vi "FanPressure2.vi"() -> ()   [LabVIEW 2023]
uses:
  <vilib>/drjdpowell/SQLite Library/SQL Connection/Connection.lvclass
  <vilib>/Instr/_visa.llb/VISA Find Search Mode.ctl
  <vilib>/drjdpowell/SQLite Library/SQL Connection/Open (path).vi
  <vilib>/Analysis/baseanly.llb/Mean (DBL).vi
  <vilib>/drjdpowell/SQLite Library/SQL Connection/Open (string).vi
  <vilib>/Instr/_visa.llb/VISA Configure Serial Port (Instr).vi
  <vilib>/drjdpowell/SQLite Library/SQL Connection/Execute SQL (No results).vi
  <vilib>/AdvancedString/Path To Command Line String.vi
  <vilib>/Analysis/NI_AALBase.lvlib
  <vilib>/drjdpowell/SQLite Library/SQLite.lvlib
panel:
  in  "Reset Plot 2":bool
  out "DC Power":bool
  in  "Message":string
  out "Receive Type":T1
  out "user event out":refnum<user-event>
  out "Table Name":string
  out "Table Created":bool
  out "time string":string
  out "date string":string
  out "SQLite Connection":refnum<class "Connection.lvclass">
  in  "View Data":bool
  in  "Reset Plot":bool
  in  "Write To Database":bool
  in  "Interval Time":u32=200
  out "Fan Speed":i32
  out "Fan Shunt Voltage":u16
  out "Fan Power":sgl
  out "Fan current":sgl
  out "Fan Voltage":sgl
  in  "Speed Control":enum32{"Values", "Paramters"}(tab)
  in  "Control Mode":enum32{"Auto", "Manual"}(radio)=enum."Manual"
  in  "Speed Setup":u16=2000 min=10 max=36 step=1
  in  "Output":sgl(knob) min=0 max=30 step=0.1 scale=0.0..30.0 scale format="%.1f"
  in  "Min Voltage":u32 max=12 step=1
  in  "Max Voltage":u32=30 min=12 max=36
  in  "Parameter Read Button":bool
  in  "Parameter Write Button":bool
  in  "Fan Speed At Full Output":u32
  in  "Fan Speed At 50% Output":u32
  in  "KD":sgl
  in  "KI":sgl=0.00015
  in  "KP":sgl=0.0024
  in  "Write Data":bool
  in  "Start Button":bool
  out "MCU":bool
  out "Serial Port":refnum<visa-resource-name>
  in  "stop":bool
  in  "Tab Control":enum32{"Readings", "Raw Data"}(tab)
  out "Waveform Chart 2":dbl[][](graph)
  out "Waveform Chart":sgl[][](graph)
  out "data":dynamicdata(graph) caption="Raw Data"
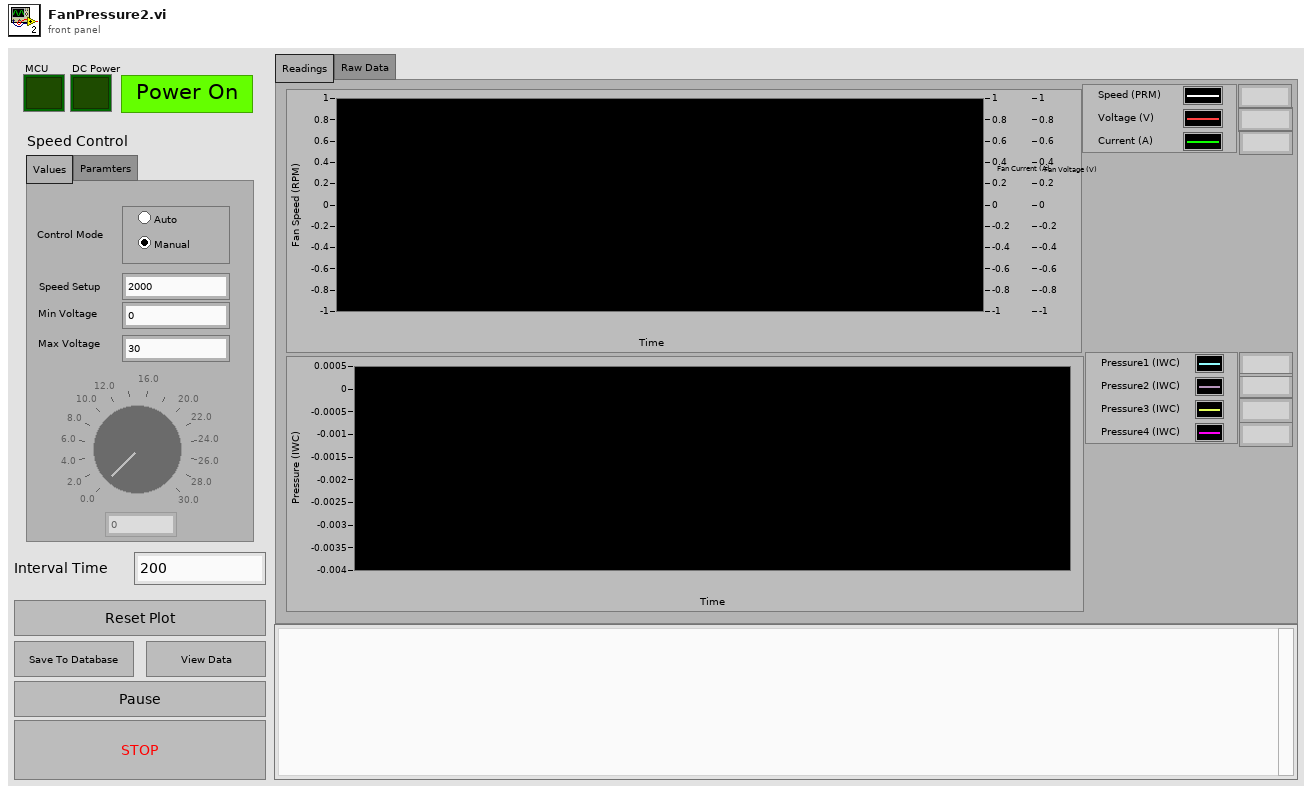
[diagram p1: front panel]
types:
  T1 = cluster{u8, u8, u8, u8, u16, u16, i16, i16, i16, i16, u16, u16, u16, u16, u16, u16, sgl, sgl, sgl, u32, u32, u8, u8, u8, u8}
  T2 = enum16{"New or existing", "Existing", "Read only"}
  T3 = enum8{"Enabled", "Disabled", "Disabled and Grayed Out"}
  T4 = enum32{"Invalid", "Standard", "Closed", "Hidden", "Minimized", "Maximized"}
  T5 = cluster{u32, "Fan current":sgl, "Fan current":sgl, "Fan current":sgl, "Fan Power":sgl, sgl, sgl, sgl, sgl, sgl, "Output":sgl, "Output":sgl}
  T6 = enum16{"big-endian, network order", "native, host order", "little-endian"}
  T7 = typedef "VISA Find Search Mode.ctl" = u32
  T8 = cluster{"y":u8, "y":u8, "y":u8, u8, u16, "Speed Setup":u16, u16, u16, "y":u8, "y":u8, "y":u8, "y":u8}
  T9 = cluster{"y":u8, "y":u8, "y":u8, "y":u8, "KP":sgl, "KI":sgl, "KD":sgl, "Fan Speed At 50% Output":u32, "Fan Speed At Full Output":u32, "y":u8, "y":u8, "y":u8, "y":u8}
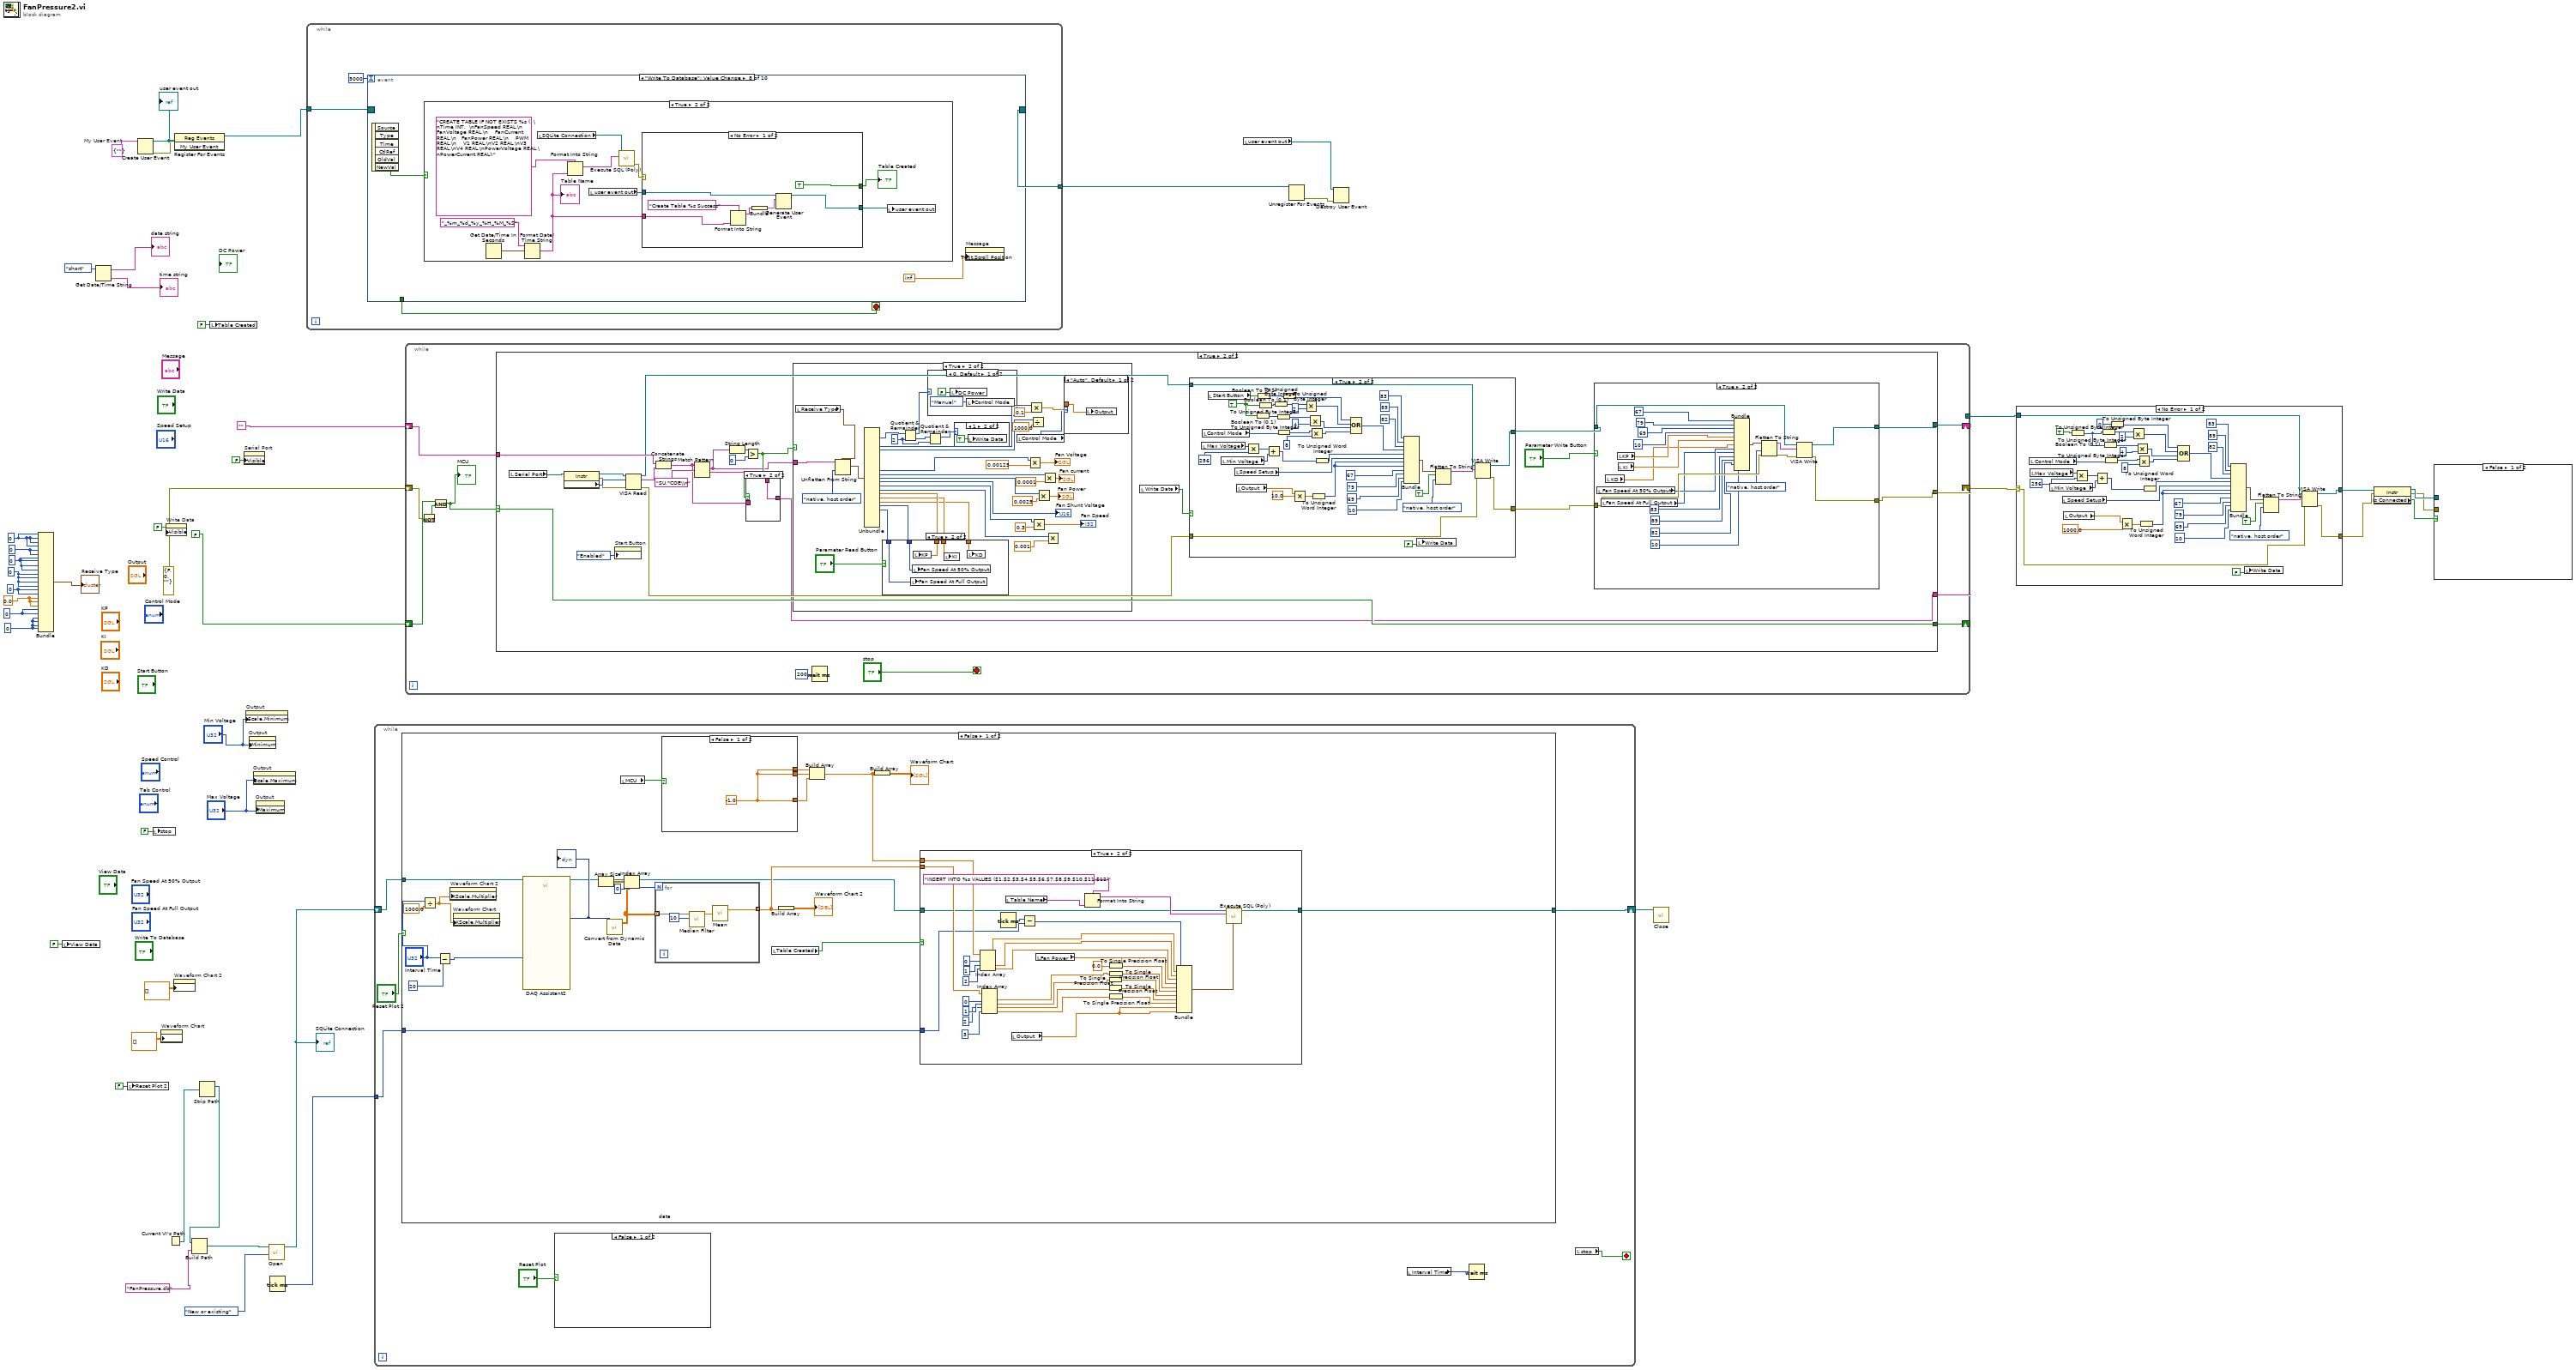
[diagram p0: block diagram]
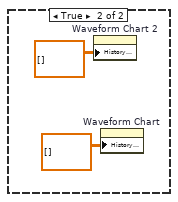
[diagram p2: hidden frame]
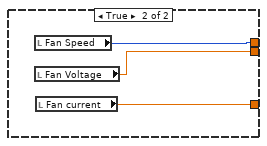
[diagram p4: hidden frame]
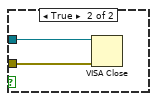
[diagram p6: hidden frame]
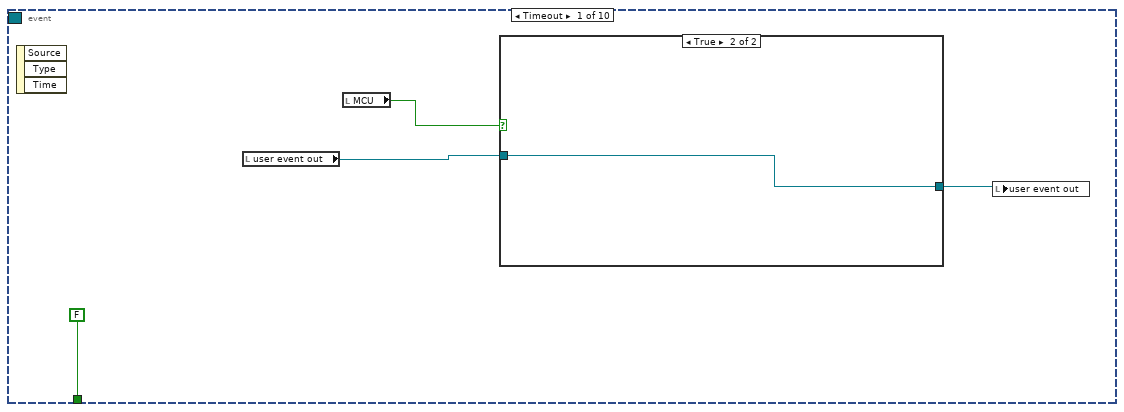
[diagram p8: hidden frame]
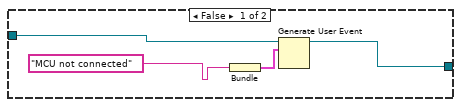
[diagram p9: hidden frame]
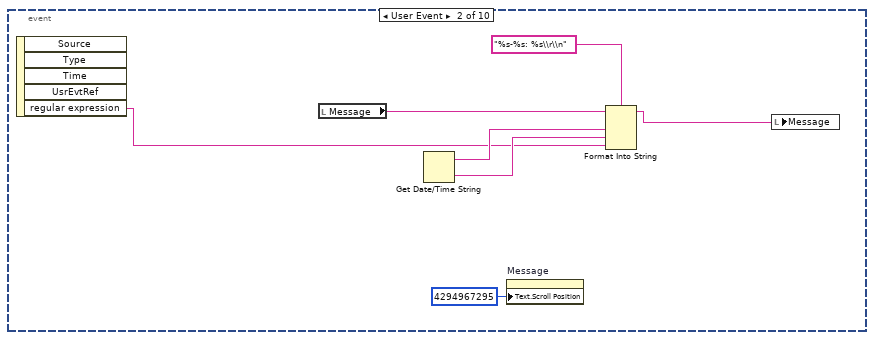
[diagram p10: hidden frame]
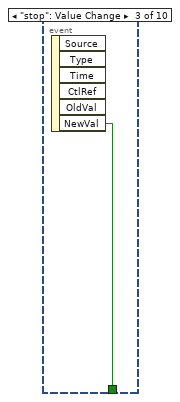
[diagram p11: hidden frame]
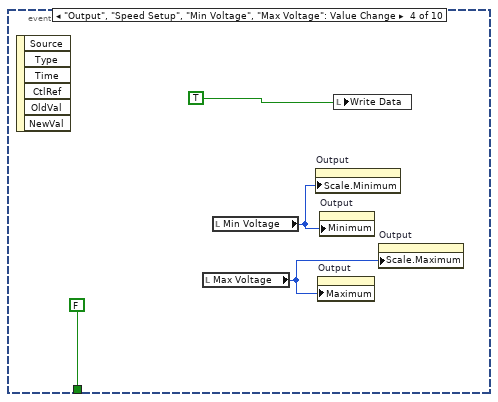
[diagram p12: hidden frame]
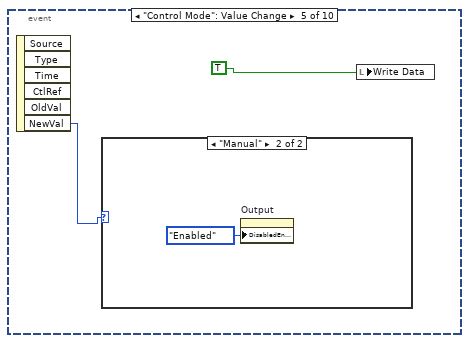
[diagram p13: hidden frame]
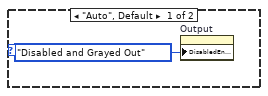
[diagram p14: hidden frame]
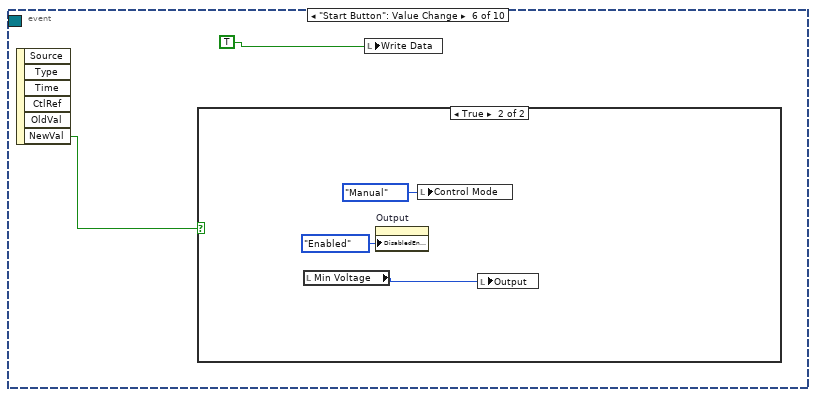
[diagram p15: hidden frame]
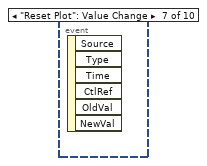
[diagram p17: hidden frame]
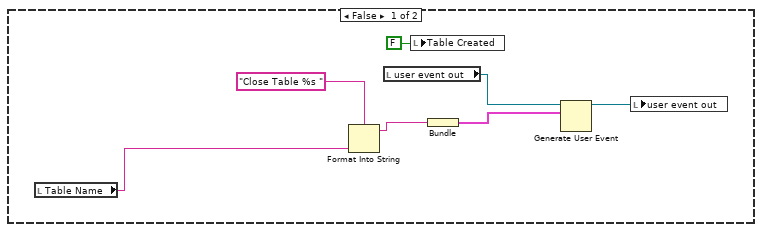
[diagram p18: hidden frame]
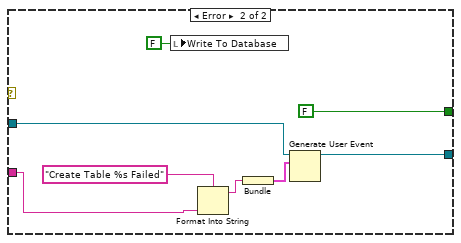
[diagram p19: hidden frame]
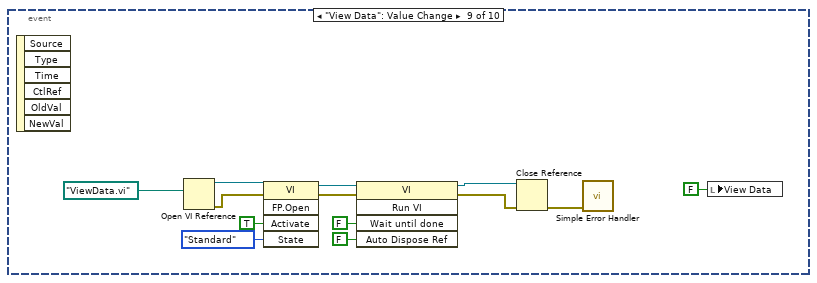
[diagram p20: hidden frame]
diagram:
  w3 = u32 0
  w4 = sgl 0.0
  w23 = cluster{"regular expression":string} {"regular expression"=""}  # My User Event
  w39 = u16 0
  w5 = u8 0
  w41 = i16 0
  w40 = u16 0
  w42 = u16 0
  w43 = u8 0
  n1 = Bundle(w43, w43, w43, w43, w42, w42, w41, w41, w41, w41, w39, w39, w39, w39, w40, w40, w4, w4, w4, w3, w3, w5, w5, w5, w5) -> (→"Receive Type":T1)  [unwired: 1 in]
  n2 = local write "View Data"(FALSE ("View Data")) -> ()
  n3 = Get Date/Time String(date format (0)=enum16{"short", "long", "abbreviated"}."short") -> (date string=→"date string":string, time string=→"time string":string)  [unwired: 2 in]
  n4 = local write "Reset Plot 2"(FALSE ("Reset Plot 2")) -> ()
  n5 = Create User Event(user event datatype=w23) -> (user event=w22:refnum<user-event>, error out=w20:errorcluster)  [unwired: 1 in]
  "user event out" <- w22
  n6 = local write "stop"(FALSE ("stop")) -> ()
  n7 = property on="Waveform Chart" class="WFChart (strict)"("History Data"=dbl[][] []) -> ()  [unwired: 2 in, 2 out]
  n8 = property on="Write Data" class="Bool (strict)"("Visible"=FALSE) -> ()  [unwired: 2 in, 2 out]
  n9 = Current VI's Path() -> (path=w14:path)
  n10 = property on="Waveform Chart 2" class="WFChart (strict)"("History Data"=dbl[][] []) -> ()  [unwired: 2 in, 2 out]
  n11 = register-events(error in=w20, w22) -> (reference out=w21:refnum<event-registration>)  [unwired: 1 in, 1 out]
  n12 = Strip Path(path=w14) -> (stripped path=w13:path)  [unwired: 1 out]
  n13 = Build Path(base path=w13, name or relative path="FanPressure.db" ("db file")) -> (appended path=w15:path)
  n14 = local write "Table Created"(FALSE ("Table Created")) -> ()
  n15 = property on="Serial Port" class="VISAName"("Visible"=FALSE) -> ()  [unwired: 2 in, 2 out]
  n16 = property on="Output" class="Knob (strict)"("Scale.Minimum"="Min Voltage") -> ()  [unwired: 2 in, 2 out]
  n17 = property on="Output" class="Knob (strict)"("Minimum"="Min Voltage") -> ()  [unwired: 2 in, 2 out]
  n18 = property on="Output" class="Knob (strict)"("Scale.Maximum"="Max Voltage") -> ()  [unwired: 2 in, 2 out]
  n19 = property on="Output" class="Knob (strict)"("Maximum"="Max Voltage") -> ()  [unwired: 2 in, 2 out]
  n20 = call-poly <vilib>:"Open.vi"("File Option"=T2."New or existing", "db file"=w15) -> ("SQLite Connection"=w12:refnum<class "Connection.lvclass">)  [unwired: 8 in, 1 out]
  "SQLite Connection" <- w12
  n21 = Tick Count (ms)() -> (millisecond timer value=w9:u32)
  n22 = while {
    tunnel: w21 -> [w50]
    tunnel: [w49] -> w19
    stop <- w51 stop-if-true
    n23 = event shown="[7] \"Write To Database\": Value Change" {
      selector: w50 -> [_ _ _ _ _ _ _ _ _ _]
      dyn-events: [_ _ _ _ _ _ _ _ _ _] -> w49
      timeout: 5000 -> [_ _ _ _ _ _ _ _ _ _]
      tunnel: [FALSE ("NewVal") _ w68 FALSE ("NewVal") _ _ _ _ _ _] -> w51
      event Timeout {
        n24 = event-data() -> ()  [unwired: 1 in, 3 out]
        n25 = local read "user event out"() -> (w54:refnum<user-event>)
        n26 = local read "MCU"() -> (w52:bool)
        n27 = case shown="True" w52 {
          tunnel: w54 -> [w57 w60]
          tunnel: [w58 w60] -> w53
          frame False {
            n28 = Bundle("format string"="MCU not connected") -> (w59:cluster{"format string":string})  [unwired: 1 in]
            n29 = Generate User Event(user event=w57, event data cluster=w59) -> (user event out=w58:refnum<user-event>)  [unwired: 2 in, 1 out]
          }
          frame True {
          }
        }
        n30 = local write "user event out"(w53) -> ()
      }
      event User Event {
        n31 = event-data() -> ("regular expression"=w62:string)  [unwired: 1 in, 4 out]
        n32 = local read "Message"() -> (w67:string)
        n33 = Get Date/Time String() -> (date string=w66:string, time string=w65:string)  [unwired: 3 in]
        n34 = property on="Message" class="Str"("Text.Scroll Position"=u32 4294967295) -> ()  [unwired: 2 in, 2 out]
        n35 = Format Into String(format string="%s-%s: %s\\r\\n", initial string=w67, w66, w65, w62) -> (resulting string=w64:string)  [unwired: 1 in, 1 out]
        n36 = local write "Message"(w64) -> ()
      }
      event "stop": Value Change {
        n37 = event-data() -> ("NewVal"=w68:bool)  [unwired: 1 in, 5 out]
      }
      event "Output", "Speed Setup", "Min Voltage", "Max Voltage": Value Change {
        n38 = event-data() -> ()  [unwired: 1 in, 6 out]
        n39 = local read "Max Voltage"() -> (w69:u32)
        n40 = local read "Min Voltage"() -> (w70:u32)
        n41 = property on="Output" class="Knob (strict)"("Scale.Minimum"=w70) -> ()  [unwired: 2 in, 2 out]
        n42 = property on="Output" class="Knob (strict)"("Maximum"=w69) -> ()  [unwired: 2 in, 2 out]
        n43 = property on="Output" class="Knob (strict)"("Minimum"=w70) -> ()  [unwired: 2 in, 2 out]
        n44 = local write "Write Data"(TRUE ("Write Data")) -> ()
        n45 = property on="Output" class="Knob (strict)"("Scale.Maximum"=w69) -> ()  [unwired: 2 in, 2 out]
      }
      event "Control Mode": Value Change {
        n46 = event-data() -> ("NewVal"=w73:enum32{"Auto", "Manual"})  [unwired: 1 in, 5 out]
        n47 = case shown="\"Manual\"" w73 {
          frame "Auto", Default {
            n48 = property on="Output" class="Knob (strict)"("DisabledEnum"=T3."Disabled and Grayed Out" ("Disabled")) -> ()  [unwired: 2 in, 2 out]
          }
          frame "Manual" {
            n49 = property on="Output" class="Knob (strict)"("DisabledEnum"=T3."Enabled" ("Disabled")) -> ()  [unwired: 2 in, 2 out]
          }
        }
        n50 = local write "Write Data"(TRUE ("Write Data")) -> ()
      }
      event "Start Button": Value Change {
        n51 = event-data() -> ("NewVal"=w77:bool)  [unwired: 1 in, 5 out]
        n52 = case shown="True" w77 {
          frame False {
          }
          frame True {
            n53 = local read "Min Voltage"() -> (w80:u32)
            n54 = property on="Output" class="Knob (strict)"("DisabledEnum"=T3."Enabled" ("Disabled")) -> ()  [unwired: 2 in, 2 out]
            n55 = local write "Control Mode"(enum32{"Auto", "Manual"}."Manual" ("Control Mode")) -> ()
            n56 = local write "Output"(w80) -> ()
          }
        }
        n57 = local write "Write Data"(TRUE ("Write Data")) -> ()
      }
      event "Reset Plot": Value Change {
        n58 = event-data() -> ()  [unwired: 1 in, 6 out]
      }
      event "Write To Database": Value Change {
        n59 = event-data() -> ("NewVal"=w83:bool)  [unwired: 1 in, 5 out]
        n60 = case shown="True" w83 {
          frame False {
            n61 = local read "Table Name"() -> (w89:string)
            n62 = Format Into String(format string="Close Table %s ", w89) -> (resulting string=w86:string)  [unwired: 2 in, 1 out]
            n63 = local read "user event out"() -> (w87:refnum<user-event>)
            n64 = local write "Table Created"(FALSE ("Table Created")) -> ()
            n65 = Bundle(w86) -> (w85:cluster{string})  [unwired: 1 in]
            n66 = Generate User Event(user event=w87, event data cluster=w85) -> (user event out=w84:refnum<user-event>)  [unwired: 2 in, 1 out]
            n67 = local write "user event out"(w84) -> ()
          }
          frame True {
            n68 = Get Date/Time In Seconds() -> (seconds since 1Jan1904=w99:timestamp)
            n69 = Format Date/Time String(time format string (%c)="_%m_%d_%y_%H_%M_%S", seconds (now)=w99) -> (date/time string=w91:string)  [unwired: 1 in]
            "Table Name" <- w91
            n70 = local read "SQLite Connection"() -> (w100:refnum<class "Connection.lvclass">)
            n71 = Format Into String(format string="CREATE TABLE IF NOT EXISTS %s (  \nTime INT,  \nFanSpeed REAL,\n    FanVoltage REAL,\n    FanCurrent REAL,\n   FanPower REAL,\n    PWM REAL,\n    V1 REAL,\nV2 REAL,\nV3 REAL,\nV4 REAL,\nPowerVoltage REAL,\nPowerCurrent REAL);" ("SQL"), w91) -> (resulting string=w96:string)  [unwired: 2 in, 1 out]
            n72 = local read "user event out"() -> (w93:refnum<user-event>)
            n73 = call-poly <vilib>:"Execute SQL (Poly).vi"("SQL"=w96, "SQLite Connection in"=w100) -> ("error out"=w95:errorcluster)  [unwired: 8 in, 1 out]
            n74 = case shown="No Error" w95 {
              tunnel: [TRUE ("Table Created") FALSE ("Table Created")] -> w94
              tunnel: w93 -> [w101 w110]
              tunnel: [w102 w109] -> w92
              tunnel: w91 -> [w103 w108]
              frame No Error {
                n75 = Format Into String(format string="Create Table %s Success", w103) -> (resulting string=w106:string)  [unwired: 2 in, 1 out]
                n76 = Bundle(w106) -> (w105:cluster{string})  [unwired: 1 in]
                n77 = Generate User Event(user event=w101, event data cluster=w105) -> (user event out=w102:refnum<user-event>)  [unwired: 2 in, 1 out]
              }
              frame Error {
                n78 = local write "Write To Database"(FALSE ("Write To Database")) -> ()
                n79 = Format Into String(format string="Create Table %s Failed", w108) -> (resulting string=w113:string)  [unwired: 2 in, 1 out]
                n80 = Bundle(w113) -> (w112:cluster{string})  [unwired: 1 in]
                n81 = Generate User Event(user event=w110, event data cluster=w112) -> (user event out=w109:refnum<user-event>)  [unwired: 2 in, 1 out]
              }
            }
            "Table Created" <- w94
            n82 = local write "user event out"(w92) -> ()
          }
        }
        n83 = property on="Message" class="Str"("Text.Scroll Position"=inf) -> ()  [unwired: 2 in, 2 out]
      }
      event "View Data": Value Change {
        n84 = event-data() -> ()  [unwired: 1 in, 6 out]
        n85 = Open VI Reference(vi path=path "ViewData.vi") -> (vi reference=w126:refnum<vi>, error out=w119:errorcluster)  [unwired: 5 in]
        n86 = invoke class="VI" method="FP.Open"(reference=w126, error in=w119, "Activate"=TRUE ("Activate?"), "State"=T4."Standard") -> (reference out=w123:refnum<vi>, error out=w122:errorcluster)  [unwired: 1 in, 3 out]
        n87 = invoke class="VI" method="Run VI"(reference=w123, error in=w122, "Wait until done"=FALSE ("Wait Until Done"), "Auto Dispose Ref"=FALSE ("Auto Dispose Reference")) -> (reference out=w118:refnum<vi>, error out=w117:errorcluster)  [unwired: 1 in, 3 out]
        n88 = Close Reference(reference=w118, error in (no error)=w117) -> (error out=w116:errorcluster)
        n89 = call <vilib>:"Simple Error Handler.vi"("error in (no error)"=w116) -> ()  [unwired: 4 in, 5 out]
        n90 = local write "View Data"(FALSE ("View Data")) -> ()
      }
      event "Message": Value Change {
        n91 = event-data() -> ()  [unwired: 1 in, 6 out]
      }
    }
  }
  n92 = while {
    shift-right: [w133] -> w11
    shift-left: w12 -> [w132]
    tunnel: w9 -> [w131]
    stop <- w135 stop-if-true
    n93 = case shown="False" "Reset Plot 2" {
      tunnel: [w140 w202] -> w133
      tunnel: w132 -> [w139 w202]
      tunnel: w131 -> [w138 _]
      frame False {
        n94 = Divide(x="Interval Time", y=1000.0) -> (x/y=w149:dbl)
        n95 = Subtract(x="Interval Time", y=u32 20) -> (x-y=w157:u32)
        n96 = property on="Waveform Chart 2" class="WFChart (strict)"("XScale.Multiplier"=w149) -> ()  [unwired: 2 in, 2 out]
        n97 = property on="Waveform Chart" class="WFChart (strict)"("XScale.Multiplier"=w149) -> ()  [unwired: 2 in, 2 out]
        n98 = call "DAQ Assistant2"("number of samples"=w157) -> ("data"=w159:dynamicdata)  [unwired: 16 in, 2 out]
        "data" <- w159
        n99 = call "Convert from Dynamic Data"("Dynamic Data Type"=w159) -> ("Array"=w156:dbl[][])  [unwired: 3 in]
        n100 = Array Size(array=w156) -> (size(s)=w155:i32[])
        n101 = local read "MCU"() -> (w148:bool)
        n102 = Index Array(array=w155, index=0) -> (element=w153:i32)
        n103 = for {
          N: w153 -> [_]
          tunnel: w156 -> [w201] mode=indexing
          tunnel: [w198] -> w143 mode=indexing
          n104 = call <vilib>:"Median Filter.vi"("left rank"=10, "X"=w201) -> ("Filtered X"=w199:dbl[])  [unwired: 8 in, 1 out]
          n105 = call-poly <vilib>:"Mean.vi"("X"=w199) -> ("mean"=w198:dbl)  [unwired: 1 out]
        }
        n106 = case shown="False" w148 {
          tunnel: [w194 w197] -> w147
          tunnel: [w194 w196] -> w146
          tunnel: [w194 w195] -> w145
          frame False {
            w194 = sgl -1.0 ("Fan current")
          }
          frame True {
            n107 = local read "Fan Speed"() -> (w195:i32)
            n108 = local read "Fan Voltage"() -> (w196:sgl)
            n109 = local read "Fan current"() -> (w197:sgl)
          }
        }
        n110 = local read "Table Created"() -> (w141:bool)
        n111 = Build Array(w143) -> (→"Waveform Chart 2":dbl[][])
        n112 = Build Array(w145, w146, w147) -> (w142:sgl[])
        n113 = Build Array(w142) -> (→"Waveform Chart":sgl[][])
        n114 = case shown="True" w141 {
          tunnel: w143 -> [_ w189]
          tunnel: w142 -> [_ w193]
          tunnel: w139 -> [w160 w176]
          tunnel: [w160 w175] -> w140
          tunnel: w138 -> [_ w164]
          frame False {
          }
          frame True {
            n115 = Index Array(array=w193, index #1=0 ("index"), index #2=1 ("index"), index #3=2 ("index")) -> (element #1=w184:sgl, element #2=w183:sgl, element #3=w182:sgl)
            n116 = Index Array(array=w189, index #1=0 ("index"), index #2=1 ("index"), index #3=2 ("index"), index #4=3 ("index")) -> (element #1=w168:dbl, element #2=w170:dbl, element #3=w172:dbl, element #4=w174:dbl)
            n117 = Tick Count (ms)() -> (millisecond timer value=w165:u32)
            n118 = local read "Table Name"() -> (w178:string)
            n119 = local read "Output"() -> (w161:sgl)
            n120 = Subtract(x=w165, y=w164) -> (x-y=w163:u32)
            n121 = local read "Fan Power"() -> (w181:sgl)
            n122 = Format Into String(format string="INSERT INTO %s VALUES ($1,$2,$3,$4,$5,$6,$7,$8,$9,$10,$11,$12)" ("SQL"), w178) -> (resulting string=w177:string)  [unwired: 2 in, 1 out]
            n123 = To Single Precision Float(number=w170) -> (single precision float=w169:sgl)
            n124 = To Single Precision Float(number=w172) -> (single precision float=w171:sgl)
            n125 = To Single Precision Float(number=sgl 0.0) -> (single precision float=w166:sgl)
            n126 = To Single Precision Float(number=w168) -> (single precision float=w167:sgl)
            n127 = To Single Precision Float(number=w174) -> (single precision float=w173:sgl)
            n128 = Bundle(w163, "Fan current"=w184, "Fan current"=w183, "Fan current"=w182, "Fan Power"=w181, w166, w167, w169, w171, w173, "Output"=w161, "Output"=w161) -> (w180:T5)  [unwired: 1 in]
            n129 = call-poly <vilib>:"Execute SQL (Poly).vi"("Parameter(s)"=w180, "SQL"=w177, "SQLite Connection in"=w176) -> ("SQLite Connection"=w175:refnum<class "Connection.lvclass">)  [unwired: 7 in, 1 out]
          }
        }
      }
      frame True {
      }
    }
    n130 = case shown="False" "Reset Plot" {
      frame False {
      }
      frame True {
        n131 = property on="Waveform Chart 2" class="WFChart (strict)"("History Data"=dbl[][] []) -> ()  [unwired: 2 in, 2 out]
        n132 = property on="Waveform Chart" class="WFChart (strict)"("History Data"=dbl[][] []) -> ()  [unwired: 2 in, 2 out]
      }
    }
    n133 = local read "Interval Time"() -> (w134:u32)
    n134 = Wait (ms)(milliseconds to wait=w134) -> ()  [unwired: 1 out]
    n135 = local read "stop"() -> (w135:bool)
  }
  n136 = while {
    shift-right: [w212] -> _
    shift-left: FALSE -> [w210]
    shift-right: [w211] -> w36
    shift-left: errorcluster {"status"=FALSE, "code"=0, "source"=""} ("error in (no error)") -> [w206]
    tunnel: [w208] -> w37
    shift-right: [w205] -> _
    shift-left: "" -> [w204]
    stop <- "stop" stop-if-true
    n137 = Not(x=w206) -> (.not. x?=w209:bool)
    n138 = And(x=w210, y=w209) -> (x .and. y?=w203:bool)
    "MCU" <- w203
    n139 = case shown="True" w203 {
      selector: w203 -> [w216 w270]
      tunnel: [w220 w270] -> w212
      tunnel: [w219 w263] -> w211
      tunnel: [w218 w265] -> w208
      tunnel: w204 -> [_ w275]
      tunnel: ["" w259] -> w205
      frame False {
        w223 = T7 2 items=["Canonical Names Only"=0, "Aliases Only"=2, "Include Matching Aliases"=3, "Include All Aliases"=4] ("Search Mode")
        n140 = local write "Start Button"(w216) -> ()
        n141 = local write "DC Power"(FALSE ("DC Power")) -> ()
        n142 = property on="Start Button" class="Bool (strict)"("DisabledEnum"=T3."Disabled and Grayed Out" ("Disabled")) -> ()  [unwired: 2 in, 2 out]
        n143 = VISA Find Resource(10:w223, 11:"ASRL[0-9]*::?*INSTR" ("expression (\"?*\")")) -> (0:w221:errorcluster, 3:w222:string[])  [unwired: 1 in, 1 out]
        n144 = for {
          tunnel: w222 -> [w229] mode=indexing
          tunnel: w221 -> [w241]
          tunnel: [w233] -> w220
          tunnel: [w226] -> w219
          tunnel: [w225] -> w218
          stop <- w232 stop-if-true
          n145 = call-poly "VISA Configure Serial Port"("VISA resource name"=w229, "baud rate (9600)"=u32 115200, "error in (no error)"=w241) -> ("VISA resource name out"=w228:refnum<visa-resource-name>, "error out"=w240:errorcluster)  [unwired: 11 in]
          n146 = property class="Instr"(reference=w228, error in=w240) -> (reference out=w231:refnum<visa-resource-name>, error out=w237:errorcluster, "Intf Inst Name"=w239:string)
          n147 = Search and Replace String(case sensitive?=TRUE ("ignore case? (F)"), input string=w239, search string="CP210x", error in=w237) -> (number of replacements=w235:i32, error out=w227:errorcluster)  [unwired: 4 in, 2 out]
          n148 = Greater?(x=w235, y=0) -> (0:w233:bool)
          n149 = case shown="True" w233 {
            selector: w233 -> [w245 w256]
            tunnel: [w245 w256] -> w232
            tunnel: w231 -> [w242 w254]
            tunnel: w227 -> [w244 w255]
            tunnel: [w243 w248] -> w226
            tunnel: [w242 w250] -> w225
            frame False {
              n150 = VISA Close(VISA resource name=w242, error in (no error)=w244) -> (error out=w243:errorcluster)
            }
            frame True {
              n151 = VISA Close(VISA resource name=w254, error in (no error)=w255) -> (error out=w247:errorcluster)
              n152 = call-poly "VISA Configure Serial Port"("VISA resource name"=w254, "baud rate (9600)"=u32 115200, "error in (no error)"=w247) -> ("VISA resource name out"=w252:refnum<visa-resource-name>, "error out"=w246:errorcluster)  [unwired: 11 in]
              n153 = VISA Open(error in (no error)=w246, VISA resource name=w252) -> (VISA resource name=w251:refnum<visa-resource-name>, error out=w249:errorcluster)  [unwired: 3 in]
              n154 = VISA Flush I/O Buffer(VISA resource name=w251, error in (no error)=w249) -> (VISA resource name out=w250:refnum<visa-resource-name>, error out=w248:errorcluster)  [unwired: 1 in]
              "Serial Port" <- w250
            }
          }
        }
      }
      frame True {
        n155 = local read "Serial Port"() -> (w280:refnum<visa-resource-name>)
        n156 = property class="Instr"(reference=w280) -> (reference out=w278:refnum<visa-resource-name>, error out=w277:errorcluster, "Serial Settings:Number of Bytes at Serial Port"=w279:u32)  [unwired: 1 in]
        n157 = property on="Start Button" class="Bool (strict)"("DisabledEnum"=T3."Enabled" ("Disabled")) -> ()  [unwired: 2 in, 2 out]
        n158 = VISA Read(VISA resource name=w278, byte count=w279, error in (no error)=w277) -> (VISA resource name out=w271:refnum<visa-resource-name>, read buffer=w276:string, error out=w267:errorcluster)  [unwired: 1 out]
        n159 = Concatenate Strings(w275, w276) -> (w258:string)
        n160 = Match Pattern(string=w258, regular expression="SU.*COE\\n") -> (match substring=w260:string, after substring=w257:string)  [unwired: 1 in, 2 out]
        n161 = String Length(string=w260) -> (length=w273:i32)
        n162 = Greater?(x=w273, y=0) -> (0:w261:bool)
        n163 = case shown="True" w261 {
          tunnel: [w281 w282] -> w259
          tunnel: w257 -> [_ w282]
          tunnel: w258 -> [w281 _]
          frame False {
          }
          frame True {
          }
        }
        n164 = case shown="True" w261 {
          tunnel: w260 -> [_ w387]
          frame False {
          }
          frame True {
            w353 = u8 2 ("y")
            n165 = local read "Receive Type"() -> (w364:T1)
            n166 = Unflatten From String(type=w364, binary string=w387, byte order (0:big-endian, network order)=T6."native, host order") -> (value=w385:T1)  [unwired: 2 in, 2 out]
            n167 = Unbundle(w385) -> (w355:u8, w384:u16, w382:u16, w379:u16, w375:u16, w373:u16, →"Fan Shunt Voltage":u16, w369:u16, w367:u16, w362:sgl, w361:sgl, w360:sgl, w359:u32, w358:u32)  [unwired: 11 out]
            n168 = case shown="True" "Parameter Read Button" {
              tunnel: w362 -> [_ w397]
              tunnel: w361 -> [_ w396]
              tunnel: w360 -> [_ w395]
              tunnel: w359 -> [_ w394]
              tunnel: w358 -> [_ w393]
              frame False {
              }
              frame True {
                n169 = local write "Fan Speed At Full Output"(w393) -> ()
                n170 = local write "Fan Speed At 50% Output"(w394) -> ()
                n171 = local write "KP"(w397) -> ()
                n172 = local write "KI"(w396) -> ()
                n173 = local write "KD"(w395) -> ()
              }
            }
            n174 = Quotient & Remainder(x=w355, y=w353) -> (x-y*floor(x/y)=w356:u8, floor(x/y)=w354:u8)
            n175 = case shown="0, Default" w356 {
              frame 0, Default {
                n176 = local write "DC Power"(FALSE ("DC Power")) -> ()
                n177 = local write "Control Mode"(enum32{"Auto", "Manual"}."Manual" ("Control Mode")) -> ()
              }
              frame 1 {
                n178 = local write "DC Power"(TRUE ("DC Power")) -> ()
              }
            }
            n179 = Quotient & Remainder(x=w354, y=w353) -> (x-y*floor(x/y)=w352:u8)  [unwired: 1 out]
            n180 = case shown="1" w352 {
              frame 0, Default {
              }
              frame 1 {
                n181 = local write "Write Data"(TRUE ("Write Data")) -> ()
              }
            }
            n182 = local read "Control Mode"() -> (w357:enum32{"Auto", "Manual"})
            n183 = Multiply(x=w379, y=0.00125) -> (x*y=→"Fan Voltage":dbl)
            n184 = Multiply(x=w384, y=0.1) -> (x*y=w365:dbl)
            n185 = Divide(x=w382, y=1000.0) -> ()  [unwired: 1 out]
            n186 = Multiply(x=w369, y=0.3) -> (x*y=→"Fan Speed":dbl)
            n187 = Multiply(x=w373, y=0.0025) -> (x*y=→"Fan Power":dbl)
            n188 = Multiply(x=w375, y=0.0001) -> (x*y=→"Fan current":dbl)
            n189 = Multiply(x=w367, y=0.001) -> ()  [unwired: 1 out]
            n190 = case shown="\"Auto\", Default" w357 {
              tunnel: w365 -> [w392 _]
              frame "Auto", Default {
                n191 = local write "Output"(w392) -> ()
              }
              frame "Manual" {
              }
            }
          }
        }
        n192 = local read "Write Data"() -> (w268:bool)
        n193 = case shown="True" w268 {
          tunnel: w271 -> [w307 w351]
          tunnel: [w307 w350] -> w266
          tunnel: w267 -> [w306 w349]
          tunnel: [w306 w348] -> w264
          frame False {
          }
          frame True {
            w314 = TRUE ("Boolean")
            n194 = local read "Max Voltage"() -> (w313:u32)
            n195 = local read "Control Mode"() -> (w315:enum32{"Auto", "Manual"})
            n196 = local read "Start Button"() -> (w344:bool)
            n197 = local read "Min Voltage"() -> (w310:u32)
            n198 = local read "Speed Setup"() -> (w328:u16)
            n199 = local read "Output"() -> (w326:sgl)
            n200 = Multiply(x=w313, y=u32 256) -> (x*y=w311:u32)
            n201 = Boolean To (0,1)(Boolean=w314) -> (0, 1=w343:i16)
            n202 = Boolean To (0,1)(Boolean=w344) -> (0, 1=w345:i16)
            n203 = Boolean To (0,1)(Boolean=w314) -> (0, 1=w346:i16)
            n204 = Add(x=w311, y=w310) -> (x+y=w309:u32)
            n205 = To Unsigned Byte Integer(number=w346) -> (unsigned 8bit integer=w338:u8)
            n206 = To Unsigned Byte Integer(number=w343) -> (unsigned 8bit integer=w335:u8)
            n207 = To Unsigned Byte Integer(number=w315) -> (unsigned 8bit integer=w334:u8)
            n208 = To Unsigned Byte Integer(number=w345) -> (unsigned 8bit integer=w342:u8)
            n209 = Multiply(x=w326, y=sgl 10.0) -> (x*y=w325:sgl)
            n210 = Multiply(x=w338, y=u8 2) -> (x*y=w336:u8)
            n211 = Multiply(x=w335, y=u8 4) -> (x*y=w330:u8)
            n212 = Multiply(x=w334, y=u8 8 ("x")) -> (x*y=w332:u8)
            n213 = To Unsigned Word Integer(number=w325) -> (unsigned 16bit integer=w324:u16)
            n214 = To Unsigned Word Integer(number=w309) -> (unsigned 16bit integer=w329:u16)
            n215 = Compound Arithmetic op=OR(w342, w336, w330, w332) -> (w341:u8)
            n216 = Bundle("y"=u8 83, "y"=u8 89, "y"=u8 82, w341, w329, "Speed Setup"=w328, w324, w324, "y"=u8 67, "y"=u8 79, "y"=u8 69, "y"=u8 10) -> (w316:T8)  [unwired: 1 in]
            n217 = local write "Write Data"(FALSE ("Write Data")) -> ()
            n218 = Flatten To String(anything=w316, prepend array or string size? (T)=TRUE, byte order (0:big-endian, network order)=T6."native, host order") -> (data string=w308:string)  [unwired: 1 in, 2 out]
            n219 = VISA Write(VISA resource name=w351, write buffer=w308, error in (no error)=w349) -> (VISA resource name out=w350:refnum<visa-resource-name>, error out=w348:errorcluster)  [unwired: 1 out]
          }
        }
        n220 = case shown="True" "Parameter Write Button" {
          tunnel: w266 -> [w284 w305]
          tunnel: [w284 w304] -> w265
          tunnel: w264 -> [w283 w301]
          tunnel: [w283 w302] -> w263
          frame False {
          }
          frame True {
            n221 = local read "Fan Speed At 50% Output"() -> (w293:u32)
            n222 = local read "Fan Speed At Full Output"() -> (w292:u32)
            n223 = local read "KD"() -> (w294:sgl)
            n224 = local read "KP"() -> (w296:sgl)
            n225 = local read "KI"() -> (w295:sgl)
            n226 = Bundle("y"=u8 67, "y"=u8 79, "y"=u8 69, "y"=u8 10, "KP"=w296, "KI"=w295, "KD"=w294, "Fan Speed At 50% Output"=w293, "Fan Speed At Full Output"=w292, "y"=u8 83, "y"=u8 89, "y"=u8 82, "y"=u8 10) -> (w287:T9)  [unwired: 1 in]
            n227 = Flatten To String(anything=w287, byte order (0:big-endian, network order)=T6."native, host order", error in (no error)=w301) -> (data string=w285:string, error out=w303:errorcluster)  [unwired: 1 in, 1 out]
            n228 = VISA Write(VISA resource name=w305, write buffer=w285, error in (no error)=w303) -> (VISA resource name out=w304:refnum<visa-resource-name>, error out=w302:errorcluster)  [unwired: 1 out]
          }
        }
      }
    }
    n229 = Wait (ms)(milliseconds to wait=u32 200) -> ()  [unwired: 1 out]
  }
  n230 = local read "user event out"() -> (w17:refnum<user-event>)
  n231 = Unregister For Events(event registration refnum=w19) -> (error out=w18:errorcluster)  [unwired: 1 in]
  n232 = Destroy User Event(user event=w17, error in=w18) -> ()  [unwired: 1 out]
  n233 = call-dynamic "Close.vi"("SQLite Connection in"=w11) -> ()  [unwired: 10 in, 1 out]
  n234 = case shown="No Error" w36 {
    selector: w36 -> [w406 w441]
    tunnel: [w439 w440] -> w34
    tunnel: [w438 w441] -> w33
    tunnel: w37 -> [w405 w440]
    frame No Error {
      n235 = local read "Control Mode"() -> (w407:enum32{"Auto", "Manual"})
      n236 = local read "Max Voltage"() -> (w402:u32)
      n237 = local read "Min Voltage"() -> (w400:u32)
      n238 = local read "Speed Setup"() -> (w422:u16)
      n239 = local read "Output"() -> (w419:sgl)
      n240 = Boolean To (0,1)(Boolean=TRUE) -> (0, 1=w403:i16)
      n241 = Multiply(x=w402, y=u32 256) -> (x*y=w401:u32)
      n242 = Add(x=w401, y=w400) -> (x+y=w398:u32)
      n243 = To Unsigned Byte Integer(number=w403) -> (unsigned 8bit integer=w432:u8)
      n244 = To Unsigned Byte Integer(number=w403) -> (unsigned 8bit integer=w429:u8)
      n245 = To Unsigned Byte Integer(number=w407) -> (unsigned 8bit integer=w428:u8)
      n246 = To Unsigned Byte Integer(number=u8 0) -> (unsigned 8bit integer=w436:u8)
      n247 = Multiply(x=w419, y=sgl 1000.0) -> (x*y=w418:sgl)
      n248 = Multiply(x=w432, y=u8 2) -> (x*y=w430:u8)
      n249 = Multiply(x=w429, y=u8 4) -> (x*y=w424:u8)
      n250 = Multiply(x=w428, y=u8 8 ("x")) -> (x*y=w426:u8)
      n251 = To Unsigned Word Integer(number=w418) -> (unsigned 16bit integer=w417:u16)
      n252 = To Unsigned Word Integer(number=w398) -> (unsigned 16bit integer=w423:u16)
      n253 = Compound Arithmetic op=OR(w436, w430, w424, w426) -> (w435:u8)
      n254 = Bundle("y"=u8 83, "y"=u8 89, "y"=u8 82, w435, w423, "Speed Setup"=w422, w417, w417, "y"=u8 67, "y"=u8 79, "y"=u8 69, "y"=u8 10) -> (w409:T8)  [unwired: 1 in]
      n255 = local write "Write Data"(FALSE ("Write Data")) -> ()
      n256 = Flatten To String(anything=w409, prepend array or string size? (T)=TRUE, byte order (0:big-endian, network order)=T6."native, host order") -> (data string=w408:string)  [unwired: 1 in, 2 out]
      n257 = VISA Write(VISA resource name=w405, write buffer=w408, error in (no error)=w406) -> (VISA resource name out=w439:refnum<visa-resource-name>, error out=w438:errorcluster)  [unwired: 1 out]
    }
    frame Error {
    }
  }
  n258 = property class="Instr"(reference=w34, error in=w33) -> (reference out=w31:refnum<visa-resource-name>, error out=w30:errorcluster, "Is Connected"=w32:bool)
  n259 = case shown="False" w32 {
    tunnel: w31 -> [_ w443]
    tunnel: w30 -> [_ w442]
    frame False {
    }
    frame True {
      n260 = VISA Close(VISA resource name=w443, error in (no error)=w442) -> ()  [unwired: 1 out]
    }
  }
